vi "TSCAN Open.vi"(0 "路径输入":path, 11 "错误输入（无错误）":errorcluster) -> (4 "路径输出":path, 8 "Connect_TSCAN_Successfully":bool, 15 "错误输出":errorcluster)   [LabVIEW 2013]
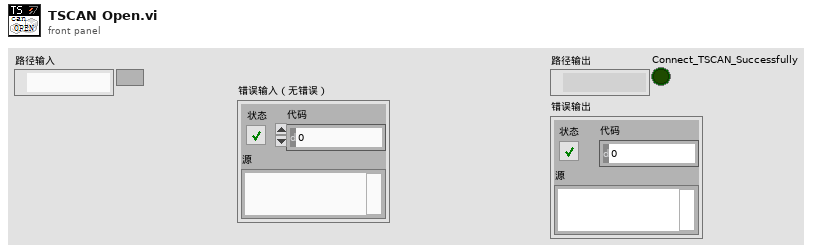
[diagram p1: front panel]
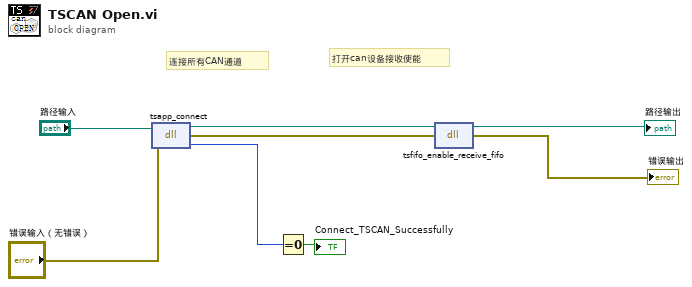
[diagram p0: block diagram]
diagram:
  # "打开can设备接收使能"
  # "连接所有CAN通道"
  n1 = dll-call lib="PTH1Habs CUsers\nAdministratorDesktopTS_Can通讯PathTSMaster.dll" fn="tsapp_connect"(path in="路径输入", error in="错误输入（无错误）") -> (path out=w6:path, error out=w1:errorcluster, "tsapp_connect"=w7:i32)  [unwired: 1 in]
  n2 = Equal To 0?(x=w7) -> (x = 0?=→"Connect_TSCAN_Successfully":bool)
  n3 = dll-call lib="PTH1Habs CUsers\nAdministratorDesktopTS_Can通讯PathTSMaster.dll" fn="tsfifo_enable_receive_fifo"(path in=w6, error in=w1) -> (path out=→"路径输出":path, error out=→"错误输出":errorcluster)  [unwired: 2 in]
